vi "Clusters.vi"(10 "Signal":T1) -> ()   [LabVIEW 2019]
panel:
  out "Sample Rate":dbl
  out "Samples":dbl[](array[numeric])
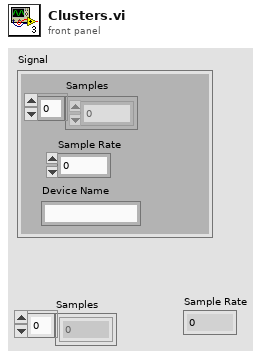
[diagram p1: front panel]
types:
  T1 = cluster{"Samples":dbl[], "Sample Rate":dbl, "Device Name":string}
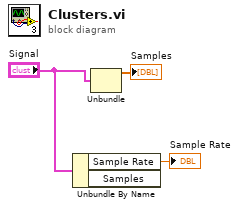
[diagram p0: block diagram]
diagram:
  n1 = Unbundle By Name("Signal") -> ("Sample Rate"=→"Sample Rate":dbl)  [unwired: 1 out]
  n2 = Unbundle("Signal") -> ("Samples"=→"Samples":dbl[])  [unwired: 2 out]
